vi "SendTrigger.vi"(8 "System Exe time":i32, 9 "Window time":i32, 11 "TimeSquares":i32) -> (3 "millisecond timer value":u32)   [LabVIEW 2020]
uses:
  Global Variables/Time_Trigger.vi
  Global Variables/Trial_Flag.vi
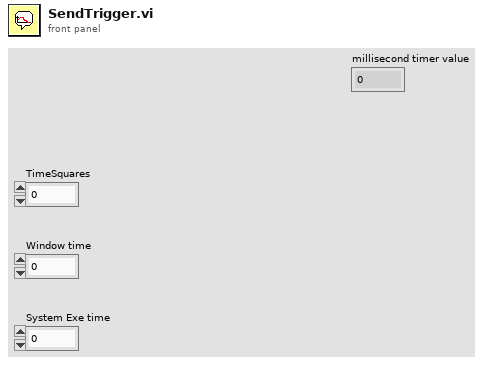
[diagram p1: front panel]
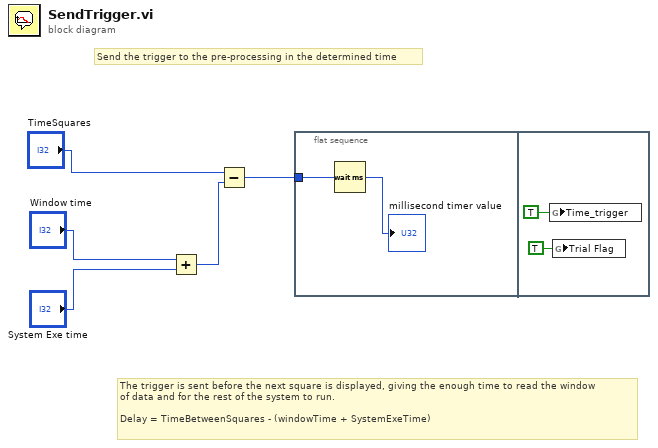
[diagram p0: block diagram]
diagram:
  # "The trigger is sent before the next square is displayed, giving the enough time to read the window \nof data and for the rest of the system to run.\n\nDelay = TimeBetweenSquares - (windowTime + SystemExeTime)"
  # "Send the trigger to the pre-processing in the determined time"
  n1 = Add(x="Window time", y="System Exe time") -> (x+y=w2:i32)
  n2 = Subtract(x="TimeSquares", y=w2) -> (x-y=w1:i32)
  n3 = flat-sequence {
    tunnel: w1 -> [w7]
    frame #0 {
      n4 = Wait (ms)(milliseconds to wait=w7) -> (millisecond timer value=→"millisecond timer value":u32)
    }
    frame #1 {
      n5 = global write "Time_Trigger.vi" "Time_trigger"(TRUE) -> ()
      n6 = global write "Trial_Flag.vi" "Trial Flag"(TRUE ("Trial Flag")) -> ()
    }
  }
